vi "Test_PIL_Main.vi"() -> ()   [LabVIEW 2015]
uses:
  controls/EXPERIMENT_Inputs.ctl
  controls/LASER_Inputs.ctl
  controls/EXPERT_Inputs.ctl
  controls/SOFTWARE_Inputs.ctl
  controls/AO_6711_Inputs.ctl
  controls/AWG_5421_Inputs.ctl
  controls/DIGIT_5122_Inputs.ctl
  <instrlib>/niScope/Controls/niScope trigger source.ctl
  controls/HSDIO_6541_Inputs.ctl
  <instrlib>/niHSDIO/niHSDIO.llb/niHSDIO_ctl Trigger Source Values (Ring).ctl
  controls/VOLTAGES_Inputs.ctl
  controls/HEXA_Inputs.ctl
  controls/QUAD_Inputs.ctl
  controls/SEQUENCE_Inputs.ctl
  controls/TRAPPING_Inputs.ctl
  controls/EXCIT_Inputs.ctl
  controls/DATA_Inputs.ctl
  controls/TIMING_Inputs.ctl
  controls/SPECTRUM.ctl
  controls/QMH_UI_Cluster.ctl
  controls/QMH_UI_References.ctl
  controls/QMH_UI_Report.ctl
  controls/QMH_UI_Command.ctl
  controls/QMH_ICR_Command.ctl
  controls/QMH_Status.ctl
panel:
  out "données":dbl format="%.2f"
  in  "error in (no error)":errorcluster
  in  "Stop":bool
  in  "Start":bool
  in  "Save":bool
  in  "Load":bool
  in  "Exit":bool
  in  "Tabs":T1(tab)
  in  "SPECTRUM":T2={"Path of the Day"=path "D:/PIRENEA/DATA/2016/data_2016_01_01", "Spectrum Name"="2016_01_01_000.A00", "Accumulated"=FALSE, "Stored in Database"=FALSE, "Record Number"=0, "Quality Flag"="Optimal"}
  in  "Change Experiment":bool
  in  "EXPERIMENT Inputs":T3={"User Name"="", "Date"="", "Comment"="", "Experiment Steps"=[], "Sample Components"=[], "Molecules"=[], "Laser 1"={"Used"=TRUE, "Name"="Spectroscopy", "Reference"="Yag", "Wavelength"=1000.0, "Energy"=25.0}, "Laser 2"={"Used"=TRUE, "Name"="Spectroscopy", "Reference"="Yag", "Wavelength"=1000.0, "Energy"=25.0}, "Laser 3"={"Used"=TRUE, "Name"="Spectroscopy", "Reference"="Yag", "Wavelength"=1000.0, "Energy"=25.0}} caption="EXCIT Paths"
  in  "Change Voltages":bool
  in  "VOLTAGES Inputs":T5={"Hexa 1"={"Used"=FALSE, "Voltage"=0.0}, "Hexa 2"={"Used"=FALSE, "Voltage"=0.0}, "Hexa 3"={"Used"=FALSE, "Voltage"=0.0}, "Quad 1"={"Used"=TRUE, "Voltage"=25.0}, "Quad 2"={"Used"=TRUE, "Voltage"=25.0}, "Quad 3"={"Used"=TRUE, "Voltage"=25.0}}
  in  "SEQUENCE Inputs":T8={"TRAPPING Inputs"={"Init Values"=[], "Opening Values"=[0.0, 0.0, 0.0, 0.0], "Trapping Values"=[2.0, 5.0, 5.0, 2.0], "Emptying Values"=[-5.0, -5.0, -5.0, -5.0], "Adiabatic ON"=FALSE, "Adiabatic Duration"=1, "Adiabatic Waveforms"=["Adiabatic_None_2_2_2000.bin", "Adiabatic_Ramp_5_0_2000.bin", "Adiabatic_DoubleRamp_5_0_2000.bin", "Adiabatic_RC_2_0_2000.bin"]}, "EXCIT Inputs"={"Number of Excitations"=1, "Table of Waveforms"=[], "Script text"=""}, "DATA Inputs"={"Record Length"=0, "Sample Rate"=enum."20", "Number of Acquisitions"=1, "Type Of Data"=enum."I16", "Vertical Range"=enum."0.2"}, "TIMING Inputs"={"Number Of Acquisitions "=1, "Number Of Accumulations"=1, "Number Of Loops"=0, "Table of Waveforms"=[], "Script text"=""}} {"TIMING Inputs"."Number Of Loops" min=0 max=10; "TIMING Inputs"."Number Of Accumulations" min=0 max=50 step=1; "TIMING Inputs"."Number Of Acquisitions" min=1 max=10 step=1; "DATA Inputs"."Number of Acquisitions" min=1 max=10; "EXCIT Inputs"."Number of Excitations" min=1 max=10; "TRAPPING Inputs"."Trapping Values" min=-10.0 max=10.0; "TRAPPING Inputs"."Init Values" min=-10.0 max=10.0; "TRAPPING Inputs"."Emptying Values" min=-10.0 max=10.0; "TRAPPING Inputs"."Opening Values" min=-10.0 max=10.0}
  in  "Change Sequence":bool
  in  "Change Expert":bool
  in  "EXPERT Inputs":T13={"SOFTWARE Inputs"={"Application Directory"=path "D:/S.O.F.T.S/LABVIEW/PIL", "Resources Path"=path "D:/S.O.F.T.S/LABVIEW/PIL/resources", "Data Path"=path "D:/PIRENEA/DATA", "XML Path"=path "D:/PIRENEA/DATA", "XML File Filter"="*.xml", "Excit Scripts Path"=path "D:/PIRENEA/EXCIT_SCRIPTS", "Excit Scripts File Filter"="*.txt", "Excit Waveforms Path"=path "D:/PIRENEA/EXCIT_WFMS", "Excit Waveforms File Filter"="*.bin", "Timing Scripts Path"=path "D:/PIRENEA/SEQUENCE_SCRIPTS", "Timing Scripts File Filter"="*.txt", "Timing Waveforms Path"=path "D:/PIRENEA/SEQUENCE_WFMS", "Timing Waveforms File Filter"="*.bin", "Trapping Waveforms Path"=path "D:/PIRENEA/TRAPPING_WFMS", "Trapping Waveforms File Filter"="*.bin"}, "AO 6711 Inputs"={"Physical Channels"="AnalogOutput/ao0:3", "Min Voltage"=-10.0, "Max Voltage"=10.0, "Trigger Source"="/AnalogOutput/PFI0", "counter"="AnalogOutput/ctr0"}, "AWG 5421 Inputs"={"Resource Name"="WaveformGenerator", "Trigger Type"=2, "Trigger Source"="PFI0", "Sample Rate"=20000000.0}, "DIGIT 5122 Inputs"={"Sample Rate"=10000000.0, "Resource Name"="Digitizer", "Channel Name"="0", "Trigger Source"="VAL_EXTERNAL", "Vertical Range"=10.0, "Trigger Level"=3.0}, "HSDIO 6541 Inputs"={"Resource Name"="SequencerHSDIO", "Clock Rate"=1000000.0, "Trigger Source"="PFI0"}} {"HSDIO 6541 Inputs"."Clock Rate" format="%.2p"; "DIGIT 5122 Inputs"."Trigger Level" format="%.2f"; "DIGIT 5122 Inputs"."Vertical Range" format="%.2f"; "DIGIT 5122 Inputs"."Sample Rate" step=1000000.0 format="%.3p"; "AWG 5421 Inputs"."Sample Rate" format="%.2p"; "AWG 5421 Inputs"."Trigger Type" items=["None", "Software Edge", "Digital Edge", "Digital Level"]; "AO 6711 Inputs"."Max Voltage" min=-10.0 max=10.0; "AO 6711 Inputs"."Min Voltage" min=-10.0 max=10.0}
  out "QMH Status":string
  out "ICR Status":string
  out "QLA Status":string
  out "UI Status":string
  # "Name"
  # "Reference"
  # "(nm)"
  # "E (J)"
  # "Laser 1"
  # "Laser 2"
  # "Laser 3"
  # "HEXAPOLE"
  # "QUADRIPOLE"
  # "Gin"
  # "GI_in"
  # "GI_out"
  # "Gout"
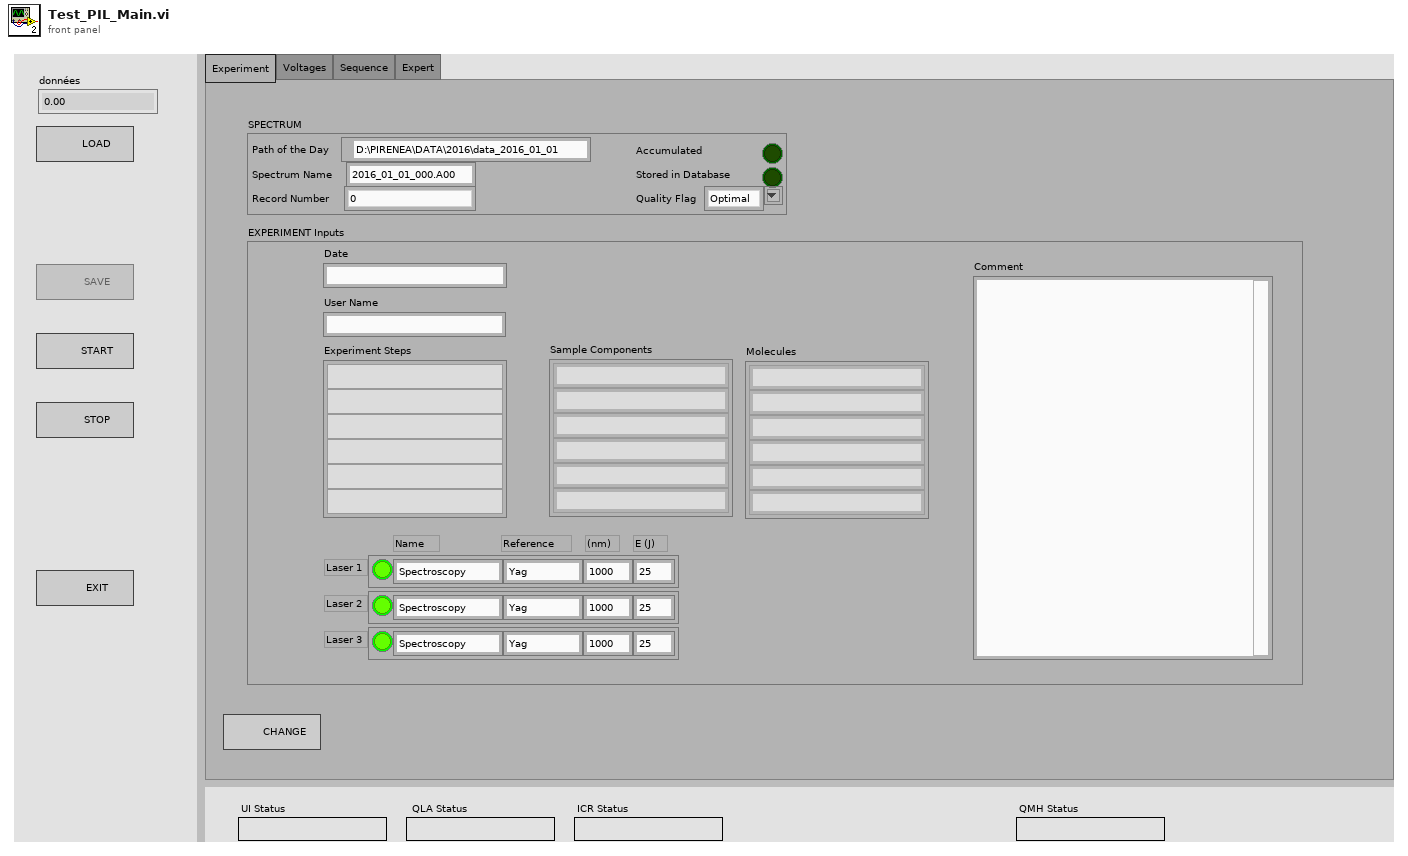
[diagram p1: front panel]
types:
  T1 = enum32{"Experiment", "Voltages", "Sequence", "Expert"}
  T2 = typedef "SPECTRUM.ctl" = cluster{"Path of the Day":path, "Spectrum Name":string, "Accumulated":bool, "Stored in Database":bool, "Record Number":i16, "Quality Flag":string}
  T3 = typedef "EXPERIMENT_Inputs.ctl" = cluster{"User Name":string, "Date":string, "Comment":string, "Experiment Steps":string[], "Sample Components":string[], "Molecules":string[], "Laser 1":T4, "Laser 2":T4, "Laser 3":T4}
  T4 = typedef "LASER_Inputs.ctl" = cluster{"Used":bool, "Name":string, "Reference":string, "Wavelength":dbl, "Energy":dbl}
  T5 = typedef "VOLTAGES_Inputs.ctl" = cluster{"Hexa 1":T6, "Hexa 2":T6, "Hexa 3":T6, "Quad 1":T7, "Quad 2":T7, "Quad 3":T7}
  T6 = typedef "HEXA_Inputs.ctl" = cluster{"Used":bool, "Voltage":dbl}
  T7 = typedef "QUAD_Inputs.ctl" = cluster{"Used":bool, "Voltage":dbl}
  T8 = typedef "SEQUENCE_Inputs.ctl" = cluster{"TRAPPING Inputs":T9, "EXCIT Inputs":T10, "DATA Inputs":T11, "TIMING Inputs":T12}
  T9 = typedef "TRAPPING_Inputs.ctl" = cluster{"Init Values":dbl[], "Opening Values":dbl[], "Trapping Values":dbl[], "Emptying Values":dbl[], "Adiabatic ON":bool, "Adiabatic Duration":i32, "Adiabatic Waveforms":string[]}
  T10 = typedef "EXCIT_Inputs.ctl" = cluster{"Number of Excitations":i32, "Table of Waveforms":string[], "Script text":string}
  T11 = typedef "DATA_Inputs.ctl" = cluster{"Record Length":i32, "Sample Rate":enum16{"1", "2", "5", "10", "20", "25", "50", "100"}, "Number of Acquisitions":i32, "Type Of Data":enum16{"I16", "DBL"}, "Vertical Range":enum16{"0.2", "0.4", "1", "2", "4", "10"}}
  T12 = typedef "TIMING_Inputs.ctl" = cluster{"Number Of Acquisitions ":i16, "Number Of Accumulations":i16, "Number Of Loops":i16, "Table of Waveforms":string[], "Script text":string}
  T13 = typedef "EXPERT_Inputs.ctl" = cluster{"SOFTWARE Inputs":T14, "AO 6711 Inputs":T15, "AWG 5421 Inputs":T16, "DIGIT 5122 Inputs":T17, "HSDIO 6541 Inputs":T19}
  T14 = typedef "SOFTWARE_Inputs.ctl" = cluster{"Application Directory":path, "Resources Path":path, "Data Path":path, "XML Path":path, "XML File Filter":string, "Excit Scripts Path":path, "Excit Scripts File Filter":string, "Excit Waveforms Path":path, "Excit Waveforms File Filter":string, "Timing Scripts Path":path, "Timing Scripts File Filter":string, "Timing Waveforms Path":path, "Timing Waveforms File Filter":string, "Trapping Waveforms Path":path, "Trapping Waveforms File Filter":string}
  T15 = typedef "AO_6711_Inputs.ctl" = cluster{"Physical Channels":tag, "Min Voltage":dbl, "Max Voltage":dbl, "Trigger Source":tag, "counter":tag}
  T16 = typedef "AWG_5421_Inputs.ctl" = cluster{"Resource Name":refnum<k15>, "Trigger Type":u16, "Trigger Source":string, "Sample Rate":dbl}
  T17 = typedef "DIGIT_5122_Inputs.ctl" = cluster{"Sample Rate":dbl, "Resource Name":refnum<k15>, "Channel Name":string, "Trigger Source":T18, "Vertical Range":dbl, "Trigger Level":dbl}
  T18 = typedef "niScope trigger source.ctl" = string
  T19 = typedef "HSDIO_6541_Inputs.ctl" = cluster{"Resource Name":refnum<k15>, "Clock Rate":dbl, "Trigger Source":T20}
  T20 = typedef "niHSDIO_ctl Trigger Source Values (Ring).ctl" = string
  T21 = typedef "QMH_UI_Cluster.ctl" = cluster{"QMH UI References":T22, "QMH UI Report":T23}
  T22 = typedef "QMH_UI_References.ctl" = cluster{"Refnum Load":refnum<vi>, "Refnum Save":refnum<vi>, "Refnum Start":refnum<vi>, "Refnum Stop":refnum<vi>, "Refnum Exit":refnum<vi>, "Refnum Tabs":refnum<vi>, "Refnum SPECTRUM":refnum<vi>, "Refnum EXPERIMENT":refnum<vi>, "Refnum VOLTAGES":refnum<vi>, "Refnum SEQUENCE":refnum<vi>, "Refnum EXPERT":refnum<vi>, "Refnum CHANGE Experiment":refnum<vi>, "Refnum CHANGE Voltages":refnum<vi>, "Refnum CHANGE Sequence":refnum<vi>, "Refnum CHANGE Expert":refnum<vi>}
  T23 = typedef "QMH_UI_Report.ctl" = cluster{"UI Status":T24, "QLA Status":string, "ICR Status":T25, "QMH Status":T26}
  T24 = typedef "QMH_UI_Command.ctl" = enum16{"Initialize", "UI Load", "UI Save", "UI Change Experiment", "UI Change Voltages", "UI Change Sequence", "UI Change Expert", "Ready to Start", "UI Start", "UI Stop", "UI Exit", "Update Report", "Update ICR Report"}
  T25 = typedef "QMH_ICR_Command.ctl" = enum16{"Initialize", "Hardware Setup", "Waiting for Trigger", "Sequence Started", "Sequence Finished", "Writing Data", "Hardware Reset", "Exit"}
  T26 = typedef "QMH_Status.ctl" = enum16{"Init", "Loading", "Setup", "Ready to Start", "Started", "Idle"}
  T27 = typedef "QMH_UI_Message.ctl" = cluster{"Command":T24, "Data":variant}
  T28 = enum32{"invalid app kind", "Development System", "Run Time System", "Student Edition", "Embedded LabVIEW", "Evaluation", "Custom"}
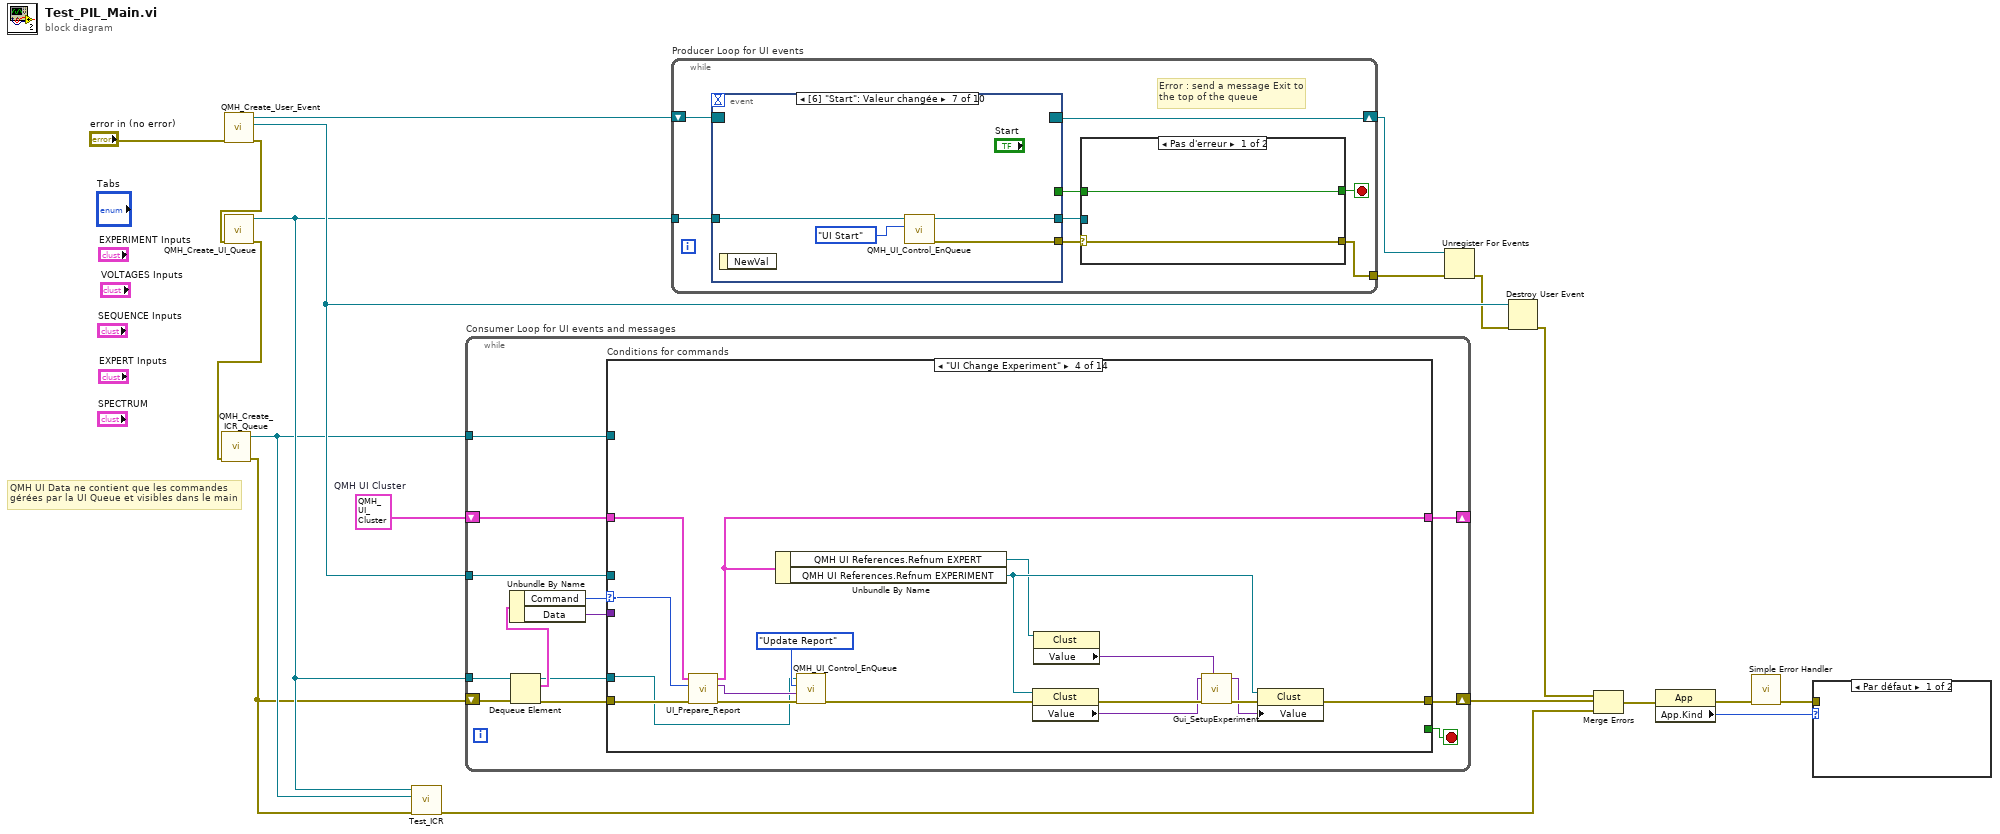
[diagram p0: block diagram]
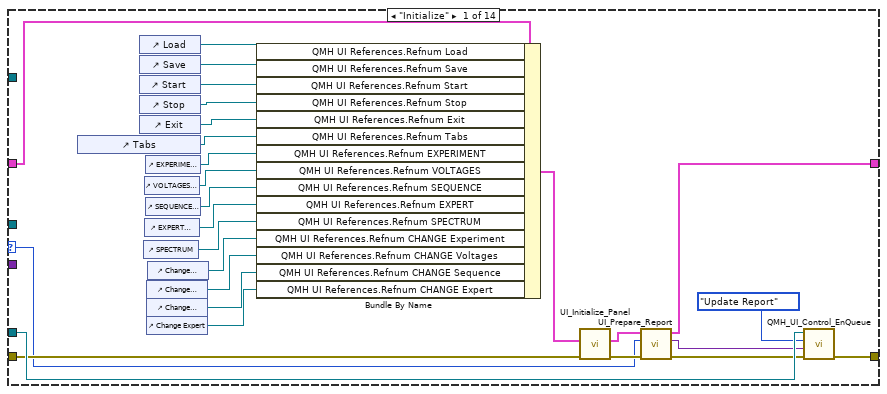
[diagram p2: hidden frame]
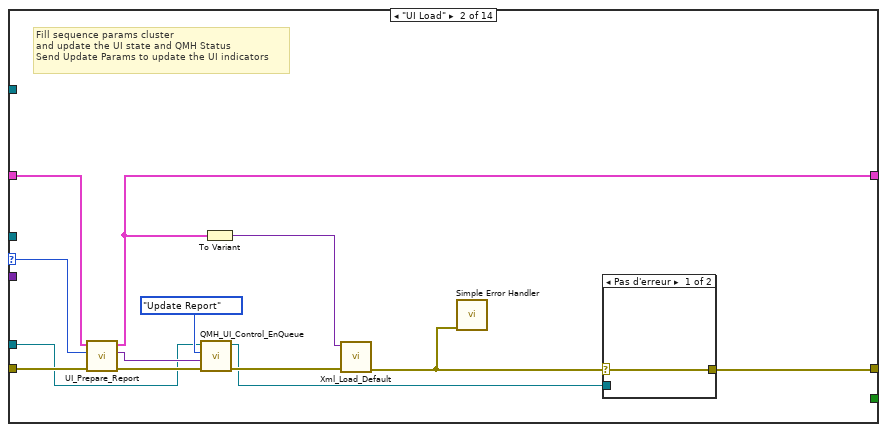
[diagram p3: hidden frame]
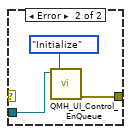
[diagram p4: hidden frame]
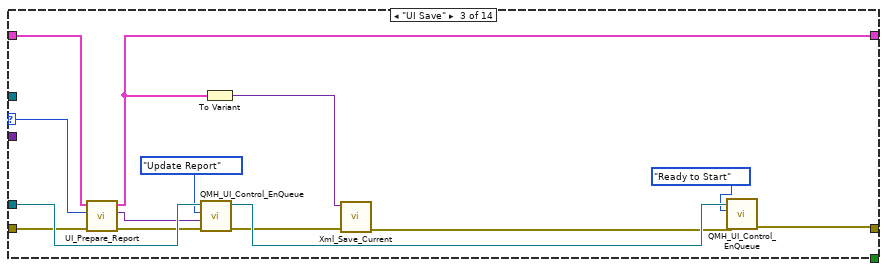
[diagram p5: hidden frame]
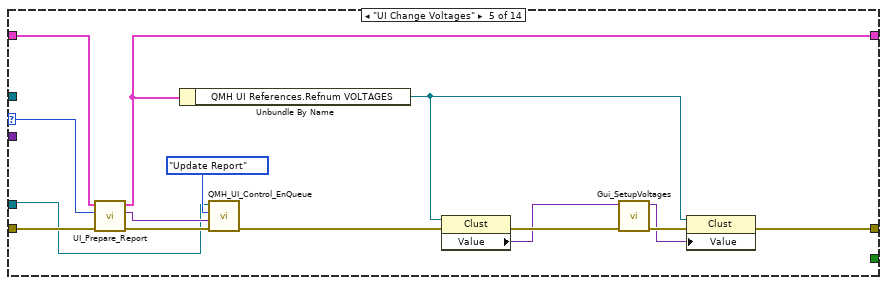
[diagram p6: hidden frame]
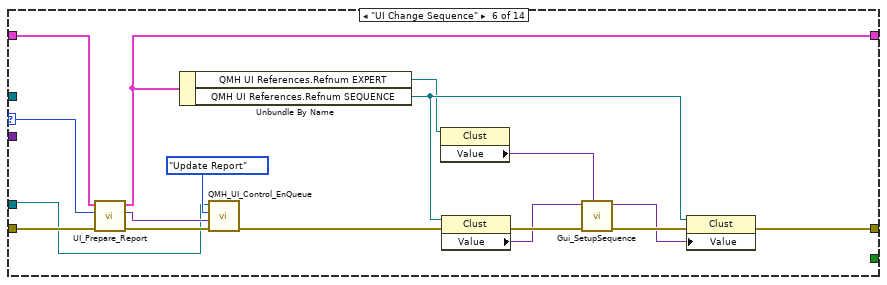
[diagram p7: hidden frame]
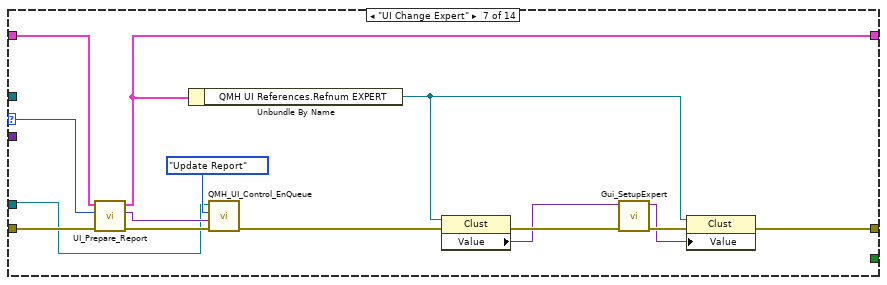
[diagram p8: hidden frame]
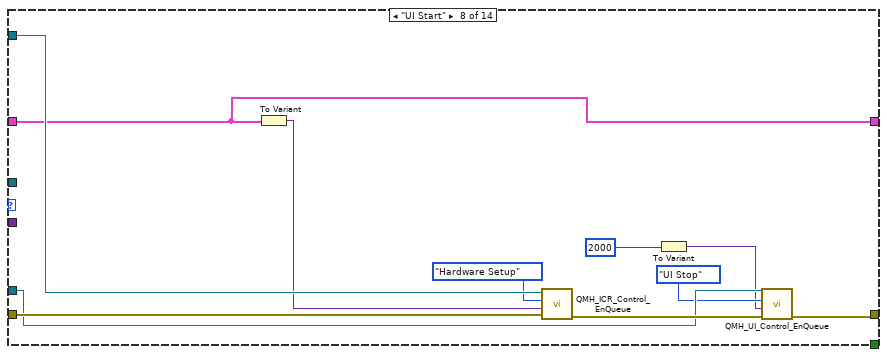
[diagram p9: hidden frame]
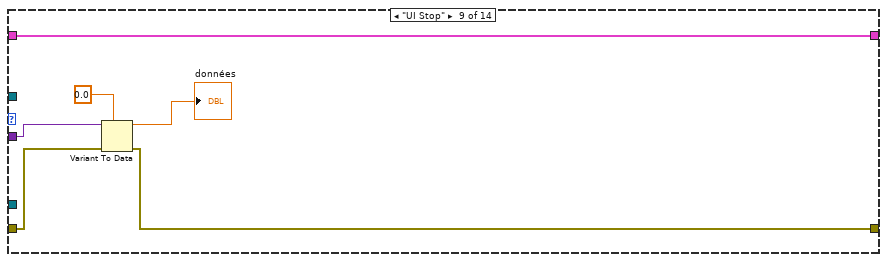
[diagram p10: hidden frame]
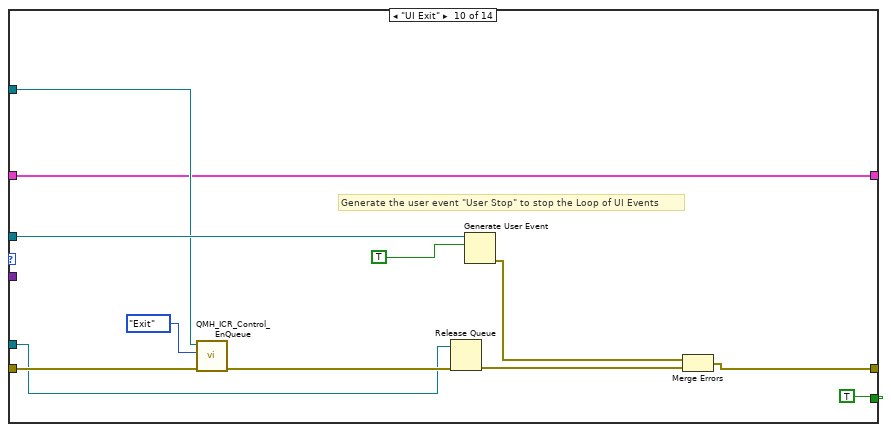
[diagram p11: hidden frame]
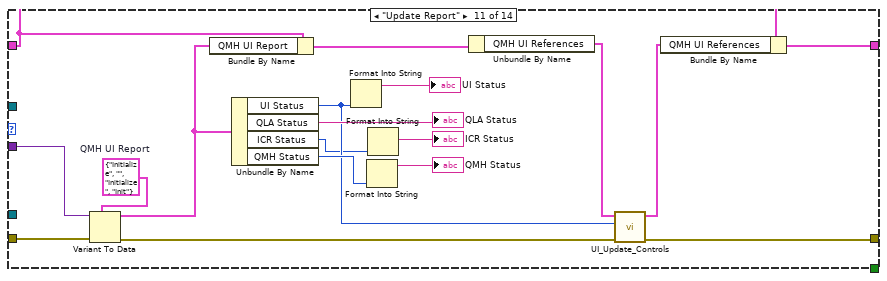
[diagram p12: hidden frame]
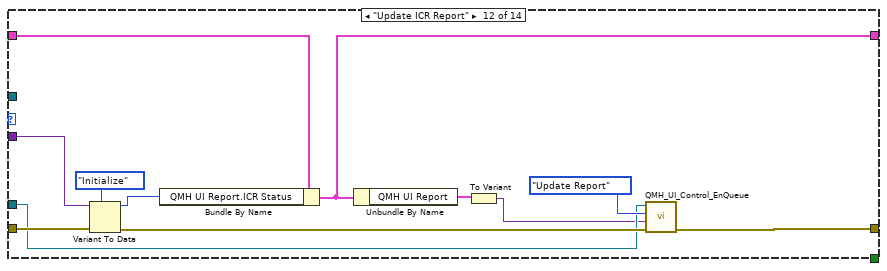
[diagram p13: hidden frame]
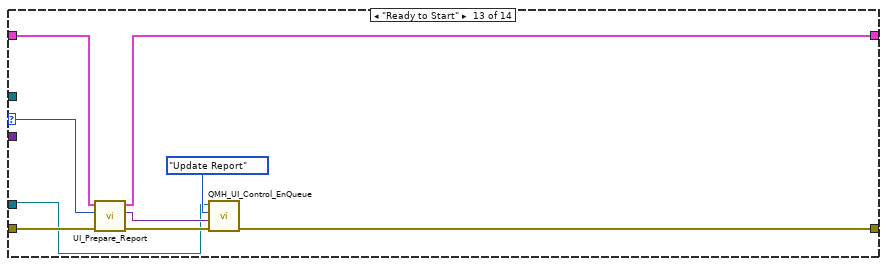
[diagram p14: hidden frame]
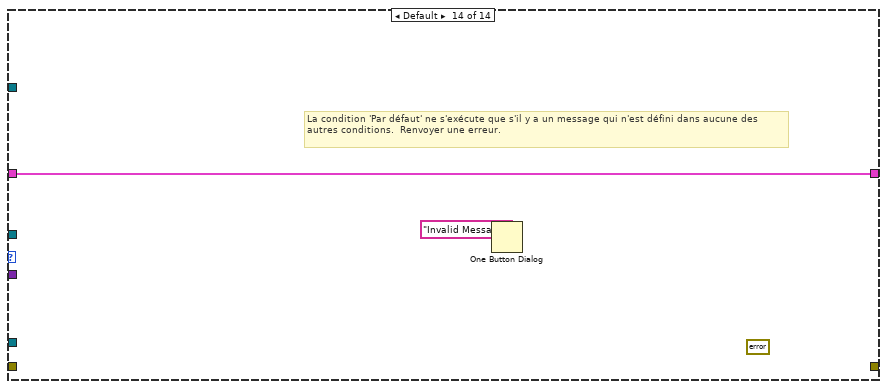
[diagram p15: hidden frame]
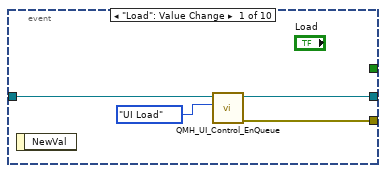
[diagram p16: hidden frame]
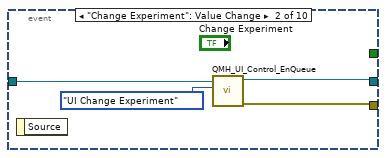
[diagram p17: hidden frame]
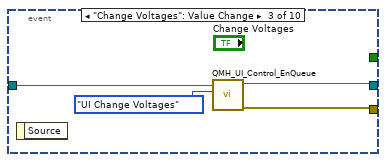
[diagram p18: hidden frame]
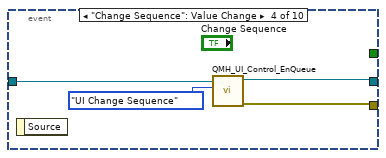
[diagram p19: hidden frame]
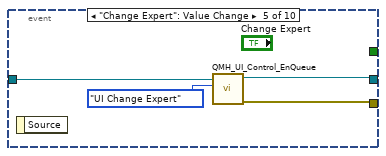
[diagram p20: hidden frame]
diagram:
  w18 = T21 {"QMH UI References"={"Refnum Load"=refnum, "Refnum Save"=refnum, "Refnum Start"=refnum, "Refnum Stop"=refnum, "Refnum Exit"=refnum, "Refnum Tabs"=refnum, "Refnum SPECTRUM"=refnum, "Refnum EXPERIMENT"=refnum, "Refnum VOLTAGES"=refnum, "Refnum SEQUENCE"=refnum, "Refnum EXPERT"=refnum, "Refnum CHANGE Experiment"=refnum, "Refnum CHANGE Voltages"=refnum, "Refnum CHANGE Sequence"=refnum, "Refnum CHANGE Expert"=refnum}, "QMH UI Report"={"UI Status"=enum."Initialize", "QLA Status"="", "ICR Status"=enum."Initialize", "QMH Status"=enum."Init"}}  # QMH UI Cluster
  # "QMH UI Data ne contient que les commandes\ngérées par la UI Queue et visibles dans le main"
  n1 = call "QMH_Create_User_Event.vi"("error in (no error)"="error in (no error)") -> ("error out"=w16:errorcluster, "User Stop Event"=w12:refnum<user-event>, "Refnum register for events"=w19:refnum<event-registration>)  [unwired: 8 in]
  n2 = call "QMH_Create_UI_Queue.vi"("error in (no error)"=w16) -> ("error out"=w2:errorcluster, "UI Queue"=w5:refnum<queue>)  [unwired: 9 in]
  n3 = call "QMH_Create_ICR_Queue.vi"("error in (no error)"=w2) -> ("error out"=w1:errorcluster, "ICR Queue"=w4:refnum<queue>)  [unwired: 9 in]
  n4 = call "Test_ICR.vi"("error in (no error)"=w1, "ICR Queue"=w4, "UI Queue"=w5) -> ("error out"=w3:errorcluster)  [unwired: 8 in]
  n5 = while "Consumer Loop for UI events and messages" {
    shift-right: [w23] -> _
    shift-left: w18 -> [w32]
    shift-right: [w21] -> w13
    shift-left: w1 -> [w28]
    tunnel: w5 -> [w29]
    tunnel: w12 -> [w24]
    tunnel: w4 -> [w20]
    stop <- w31 stop-if-true
    n6 = Dequeue Element(queue=w29, error in (no error)=w28) -> (queue out=w27:refnum<queue>, element=w30:T27, error out=w22:errorcluster)  [unwired: 2 out]
    n7 = Unbundle By Name(w30) -> ("Command"=w26:T24, "Data"=w25:variant)
    n8 = case "Conditions for commands" shown="\"UI Change Experiment\"" w26 {
      selector: w26 -> [w39 w69 w86 w102 w117 w134 w149 _ _ _ _ _ w218 _]
      tunnel: w27 -> [w53 w62 w90 w100 w115 w132 w147 w161 _ w174 _ w205 w216 _]
      tunnel: w32 -> [w54 w68 w85 w103 w118 w135 w150 w157 w166 w172 w186 w211 w219 w223]
      tunnel: [_ _ _ _ _ _ _ _ _ TRUE _ _ _ _] -> w31
      tunnel: w25 -> [_ _ _ _ _ _ _ _ w171 _ w201 w213 _ _]
      tunnel: w24 -> [_ _ _ _ _ _ _ _ _ w180 _ _ _ _]
      tunnel: [w40 w65 w79 w99 w114 w131 w146 w157 w166 w172 w196 w202 w215 w223] -> w23
      tunnel: w22 -> [w45 w70 w87 w101 w116 w133 w148 w165 w168 w176 w193 w212 w217 _]
      tunnel: [w38 w63 w82 w91 w108 w125 w140 w162 w167 w178 w192 w206 w214 _] -> w21
      tunnel: w20 -> [_ _ _ _ _ _ _ w164 _ w173 _ _ _ _]
      frame "Initialize" {
        n9 = control-ref of="Tabs"() -> (w50:refnum<vi>)
        n10 = control-ref of="Load"() -> (w59:refnum<vi>)
        n11 = control-ref of="Save"() -> (w58:refnum<vi>)
        n12 = control-ref of="Start"() -> (w57:refnum<vi>)
        n13 = control-ref of="Stop"() -> (w56:refnum<vi>)
        n14 = control-ref of="Exit"() -> (w55:refnum<vi>)
        n15 = control-ref of="SPECTRUM"() -> (w37:refnum<vi>)
        n16 = control-ref of="VOLTAGES Inputs"() -> (w48:refnum<vi>)
        n17 = control-ref of="EXPERT Inputs"() -> (w46:refnum<vi>)
        n18 = control-ref of="EXPERIMENT Inputs"() -> (w49:refnum<vi>)
        n19 = control-ref of="SEQUENCE Inputs"() -> (w47:refnum<vi>)
        n20 = control-ref of="Change Voltages"() -> (w33:refnum<vi>)
        n21 = control-ref of="Change Sequence"() -> (w34:refnum<vi>)
        n22 = control-ref of="Change Expert"() -> (w35:refnum<vi>)
        n23 = control-ref of="Change Experiment"() -> (w36:refnum<vi>)
        n24 = Bundle By Name(cluster=w54, "QMH UI References.Refnum Load"=w59, "QMH UI References.Refnum Save"=w58, "QMH UI References.Refnum Start"=w57, "QMH UI References.Refnum Stop"=w56, "QMH UI References.Refnum Exit"=w55, "QMH UI References.Refnum Tabs"=w50, "QMH UI References.Refnum EXPERIMENT"=w49, "QMH UI References.Refnum VOLTAGES"=w48, "QMH UI References.Refnum SEQUENCE"=w47, "QMH UI References.Refnum EXPERT"=w46, "QMH UI References.Refnum SPECTRUM"=w37, "QMH UI References.Refnum CHANGE Experiment"=w36, "QMH UI References.Refnum CHANGE Voltages"=w33, "QMH UI References.Refnum CHANGE Sequence"=w34, "QMH UI References.Refnum CHANGE Expert"=w35) -> (w51:T21)
        n25 = call "UI_Initialize_Panel.vi"("error in (no error)"=w45, "QMH UI Cluster"=w51) -> ("error out"=w44:errorcluster, "QMH UI Cluster"=w41:T21)  [unwired: 8 in]
        n26 = call "UI_Prepare_Report.vi"("error in (no error)"=w44, "UI Status"=w39, "QMH UI Cluster"=w41) -> ("error out"=w43:errorcluster, "Variant"=w42:variant, "QMH UI Cluster"=w40:T21)  [unwired: 6 in]
        n27 = call "QMH_UI_Control_EnQueue.vi"("error in (no error)"=w43, "Variant"=w42, "Command"=QMH_UI_Command."Update Report", "UI Queue"=w53) -> ("error out"=w38:errorcluster)  [unwired: 6 in, 1 out]
      }
      frame "UI Load" {
        # "Fill sequence params cluster\nand update the UI state and QMH Status\nSend Update Params to update the UI indicators"
        n28 = call "UI_Prepare_Report.vi"("error in (no error)"=w70, "UI Status"=w69, "QMH UI Cluster"=w68) -> ("error out"=w71:errorcluster, "Variant"=w67:variant, "QMH UI Cluster"=w65:T21)  [unwired: 6 in]
        n29 = call "QMH_UI_Control_EnQueue.vi"("error in (no error)"=w71, "Variant"=w67, "Command"=QMH_UI_Command."Update Report", "UI Queue"=w62) -> ("error out"=w66:errorcluster, "UI Queue"=w61:refnum<queue>)  [unwired: 6 in]
        n30 = To Variant(anything=w65) -> (Variant=w64:variant)
        n31 = call "Xml_Load_Default.vi"("error in (no error)"=w66, "Variant"=w64) -> ("error out"=w60:errorcluster)  [unwired: 9 in]
        n32 = call <vilib>:"Simple Error Handler.vi"("error in (no error)"=w60) -> ()  [unwired: 4 in, 5 out]
        n33 = case shown="Pas d'erreur" w60 {
          selector: w60 -> [w73 _]
          tunnel: [w73 w76] -> w63
          tunnel: w61 -> [_ w74]
          frame No Error {
          }
          frame Error {
            n34 = call "QMH_UI_Control_EnQueue.vi"("Command"=QMH_UI_Command."Initialize", "UI Queue"=w74) -> ("error out"=w76:errorcluster)  [unwired: 8 in, 1 out]
          }
        }
      }
      frame "UI Save" {
        n35 = call "UI_Prepare_Report.vi"("error in (no error)"=w87, "UI Status"=w86, "QMH UI Cluster"=w85) -> ("error out"=w88:errorcluster, "Variant"=w84:variant, "QMH UI Cluster"=w79:T21)  [unwired: 6 in]
        n36 = call "QMH_UI_Control_EnQueue.vi"("error in (no error)"=w88, "Variant"=w84, "Command"=QMH_UI_Command."Update Report", "UI Queue"=w90) -> ("error out"=w80:errorcluster, "UI Queue"=w83:refnum<queue>)  [unwired: 6 in]
        n37 = To Variant(anything=w79) -> (Variant=w78:variant)
        n38 = call "Xml_Save_Current.vi"("error in (no error)"=w80, "Variant"=w78) -> ("error out"=w77:errorcluster)  [unwired: 9 in]
        n39 = call "QMH_UI_Control_EnQueue.vi"("error in (no error)"=w77, "Command"=QMH_UI_Command."Ready to Start", "UI Queue"=w83) -> ("error out"=w82:errorcluster)  [unwired: 7 in, 1 out]
      }
      frame "UI Change Experiment" {
        n40 = call "UI_Prepare_Report.vi"("error in (no error)"=w101, "UI Status"=w102, "QMH UI Cluster"=w103) -> ("error out"=w105:errorcluster, "Variant"=w104:variant, "QMH UI Cluster"=w99:T21)  [unwired: 6 in]
        n41 = Unbundle By Name(w99) -> ("QMH UI References.Refnum EXPERT"=w93:refnum<vi>, "QMH UI References.Refnum EXPERIMENT"=w98:refnum<vi>)
        n42 = call "QMH_UI_Control_EnQueue.vi"("error in (no error)"=w105, "Variant"=w104, "Command"=QMH_UI_Command."Update Report", "UI Queue"=w100) -> ("error out"=w97:errorcluster)  [unwired: 6 in, 1 out]
        n43 = property class="Clust"(reference=w98, error in=w97) -> (error out=w96:errorcluster, "Value"=w95:variant)  [unwired: 1 out]
        n44 = property class="Clust"(reference=w93) -> ("Value"=w92:variant)  [unwired: 1 in, 2 out]
        n45 = call "Gui_SetupExperiment.vi"("Variant for Path"=w92, "error in (no error)"=w96, "Variant"=w95) -> ("error out"=w107:errorcluster, "Variant Output"=w94:variant)  [unwired: 7 in]
        n46 = property class="Clust"(reference=w98, error in=w107, "Value"=w94) -> (error out=w91:errorcluster)  [unwired: 1 out]
      }
      frame "UI Change Voltages" {
        n47 = call "UI_Prepare_Report.vi"("error in (no error)"=w116, "UI Status"=w117, "QMH UI Cluster"=w118) -> ("error out"=w120:errorcluster, "Variant"=w119:variant, "QMH UI Cluster"=w114:T21)  [unwired: 6 in]
        n48 = Unbundle By Name(w114) -> ("QMH UI References.Refnum VOLTAGES"=w113:refnum<vi>)
        n49 = call "QMH_UI_Control_EnQueue.vi"("error in (no error)"=w120, "Variant"=w119, "Command"=QMH_UI_Command."Update Report", "UI Queue"=w115) -> ("error out"=w112:errorcluster)  [unwired: 6 in, 1 out]
        n50 = property class="Clust"(reference=w113, error in=w112) -> (error out=w111:errorcluster, "Value"=w110:variant)  [unwired: 1 out]
        n51 = call "Gui_SetupVoltages.vi"("error in (no error)"=w111, "Variant"=w110) -> ("error out"=w122:errorcluster, "Variant Output"=w109:variant)  [unwired: 8 in]
        n52 = property class="Clust"(reference=w113, error in=w122, "Value"=w109) -> (error out=w108:errorcluster)  [unwired: 1 out]
      }
      frame "UI Change Sequence" {
        n53 = call "UI_Prepare_Report.vi"("error in (no error)"=w133, "UI Status"=w134, "QMH UI Cluster"=w135) -> ("error out"=w137:errorcluster, "Variant"=w136:variant, "QMH UI Cluster"=w131:T21)  [unwired: 6 in]
        n54 = Unbundle By Name(w131) -> ("QMH UI References.Refnum EXPERT"=w124:refnum<vi>, "QMH UI References.Refnum SEQUENCE"=w130:refnum<vi>)
        n55 = call "QMH_UI_Control_EnQueue.vi"("error in (no error)"=w137, "Variant"=w136, "Command"=QMH_UI_Command."Update Report", "UI Queue"=w132) -> ("error out"=w129:errorcluster)  [unwired: 6 in, 1 out]
        n56 = property class="Clust"(reference=w124) -> ("Value"=w123:variant)  [unwired: 1 in, 2 out]
        n57 = property class="Clust"(reference=w130, error in=w129) -> (error out=w128:errorcluster, "Value"=w127:variant)  [unwired: 1 out]
        n58 = call "Gui_SetupSequence.vi"("Variant For Path"=w123, "error in (no error)"=w128, "Variant"=w127) -> ("error out"=w139:errorcluster, "Variant Output"=w126:variant)  [unwired: 7 in]
        n59 = property class="Clust"(reference=w130, error in=w139, "Value"=w126) -> (error out=w125:errorcluster)  [unwired: 1 out]
      }
      frame "UI Change Expert" {
        n60 = call "UI_Prepare_Report.vi"("error in (no error)"=w148, "UI Status"=w149, "QMH UI Cluster"=w150) -> ("error out"=w152:errorcluster, "Variant"=w151:variant, "QMH UI Cluster"=w146:T21)  [unwired: 6 in]
        n61 = Unbundle By Name(w146) -> ("QMH UI References.Refnum EXPERT"=w145:refnum<vi>)
        n62 = call "QMH_UI_Control_EnQueue.vi"("error in (no error)"=w152, "Variant"=w151, "Command"=QMH_UI_Command."Update Report", "UI Queue"=w147) -> ("error out"=w144:errorcluster)  [unwired: 6 in, 1 out]
        n63 = property class="Clust"(reference=w145, error in=w144) -> (error out=w143:errorcluster, "Value"=w142:variant)  [unwired: 1 out]
        n64 = call "Gui_SetupExpert.vi"("error in (no error)"=w143, "Variant"=w142) -> ("error out"=w154:errorcluster, "Variant Output"=w141:variant)  [unwired: 8 in]
        n65 = property class="Clust"(reference=w145, error in=w154, "Value"=w141) -> (error out=w140:errorcluster)  [unwired: 1 out]
      }
      frame "UI Start" {
        n66 = To Variant(anything=w157) -> (Variant=w155:variant)
        n67 = call "QMH_ICR_Control_EnQueue.vi"("error in (no error)"=w165, "Variant"=w155, "Command"=QMH_ICR_Command."Hardware Setup", "ICR Queue"=w164) -> ("error out"=w163:errorcluster)  [unwired: 6 in, 1 out]
        n68 = To Variant(anything=2000) -> (Variant=w159:variant)
        n69 = call "QMH_UI_Control_EnQueue.vi"("error in (no error)"=w163, "Variant"=w159, "Command"=QMH_UI_Command."UI Stop", "UI Queue"=w161) -> ("error out"=w162:errorcluster)  [unwired: 6 in, 1 out]
      }
      frame "UI Stop" {
        n70 = Variant To Data(error in=w168, type=0.0, Variant=w171) -> (data=→"données":dbl, error out=w167:errorcluster)
      }
      frame "UI Exit" {
        # "Generate the user event \"User Stop\" to stop the Loop of UI Events"
        n71 = call "QMH_ICR_Control_EnQueue.vi"("error in (no error)"=w176, "Command"=QMH_ICR_Command."Exit", "ICR Queue"=w173) -> ("error out"=w175:errorcluster)  [unwired: 7 in, 1 out]
        n72 = Release Queue(queue=w174, error in (no error)=w175) -> (error out=w182:errorcluster)  [unwired: 1 in, 2 out]
        n73 = Generate User Event(user event=w180, event data cluster=TRUE ("données d'événement")) -> (error out=w179:errorcluster)  [unwired: 2 in, 1 out]
        n74 = Merge Errors(w179, w182) -> (w178:errorcluster)
      }
      frame "Update Report" {
        w200 = T23 {"UI Status"=enum."Initialize", "QLA Status"="", "ICR Status"=enum."Initialize", "QMH Status"=enum."Init"}  # QMH UI Report
        n75 = Variant To Data(error in=w193, type=w200, Variant=w201) -> (data=w188:T23, error out=w198:errorcluster)
        n76 = Bundle By Name(cluster=w186, "QMH UI Report"=w188) -> (w187:T21)
        n77 = Unbundle By Name(w188) -> ("UI Status"=w190:T24, "QLA Status"=→"QLA Status":string, "ICR Status"=w185:T25, "QMH Status"=w194:T26)
        n78 = Format Into String ("Format to String")(w190) -> (resulting string=→"UI Status":string)  [unwired: 3 in, 1 out]
        n79 = Format Into String ("Format to String")(w194) -> (resulting string=→"QMH Status":string)  [unwired: 3 in, 1 out]
        n80 = Format Into String ("Format to String")(w185) -> (resulting string=→"ICR Status":string)  [unwired: 3 in, 1 out]
        n81 = Unbundle By Name(w187) -> ("QMH UI References"=w189:T22)
        n82 = call "UI_Update_Controls.vi"("error in (no error)"=w198, "UI Status"=w190, "QMH UI References"=w189) -> ("error out"=w192:errorcluster, "QMH UI References"=w197:T22)  [unwired: 7 in]
        n83 = Bundle By Name(cluster=w186, "QMH UI References"=w197) -> (w196:T21)
      }
      frame "Update ICR Report" {
        n84 = Variant To Data(error in=w212, type=QMH_ICR_Command."Initialize" ("Command"), Variant=w213) -> (data=w209:T25, error out=w207:errorcluster)
        n85 = Bundle By Name(cluster=w211, "QMH UI Report.ICR Status"=w209) -> (w202:T21)
        n86 = Unbundle By Name(w202) -> ("QMH UI Report"=w203:T23)
        n87 = To Variant(anything=w203) -> (Variant=w204:variant)
        n88 = call "QMH_UI_Control_EnQueue.vi"("error in (no error)"=w207, "Variant"=w204, "Command"=QMH_UI_Command."Update Report", "UI Queue"=w205) -> ("error out"=w206:errorcluster)  [unwired: 6 in, 1 out]
      }
      frame "Ready to Start" {
        n89 = call "UI_Prepare_Report.vi"("error in (no error)"=w217, "UI Status"=w218, "QMH UI Cluster"=w219) -> ("error out"=w221:errorcluster, "Variant"=w220:variant, "QMH UI Cluster"=w215:T21)  [unwired: 6 in]
        n90 = call "QMH_UI_Control_EnQueue.vi"("error in (no error)"=w221, "Variant"=w220, "Command"=QMH_UI_Command."Update Report", "UI Queue"=w216) -> ("error out"=w214:errorcluster)  [unwired: 6 in, 1 out]
      }
      frame Default {
        (unwired) errorcluster {"status"=FALSE, "code"=0, "source"=""} ("sortie d'erreur")
        # "La condition 'Par défaut' ne s'exécute que s'il y a un message qui n'est défini dans aucune des autres conditions.  Renvoyer une erreur."
        n91 = One Button Dialog(message="Invalid Message") -> ()  [unwired: 1 in, 1 out]
      }
    }
  }
  n92 = while "Producer Loop for UI events" {
    tunnel: w5 -> [w231]
    tunnel: [w225] -> w15
    shift-right: [w227] -> w14
    shift-left: w19 -> [w228]
    stop <- w232 stop-if-true
    # "Error : send a message Exit to\nthe top of the queue"
    n93 = event shown="[6] \"Start\": Valeur changée" {
      selector: w228 -> [_ _ _ _ _ _ _ _ _ _]
      dyn-events: [_ _ _ _ _ _ _ _ _ _] -> w227
      timeout: _ -> [_ _ _ _ _ _ _ _ _ _]
      tunnel: w231 -> [w235 w237 w241 w245 w249 w255 w259 w263 w268 w270]
      tunnel: [w233 w238 w242 w246 w250 w253 w257 w261 w267 _] -> w230
      tunnel: [w234 w239 w243 w247 w251 w254 w258 w262 w266 w270] -> w229
      tunnel: [_ _ _ _ _ _ _ _ _ TRUE ("User Stop")] -> w226
      event "Load": Value Change {
        n94 = event-data() -> ()  [unwired: 2 out]
        n95 = call "QMH_UI_Control_EnQueue.vi"("Command"=QMH_UI_Command."UI Load", "UI Queue"=w235) -> ("error out"=w233:errorcluster, "UI Queue"=w234:refnum<queue>)  [unwired: 8 in]
      }
      event "Change Experiment": Value Change {
        n96 = event-data() -> ()  [unwired: 2 out]
        n97 = call "QMH_UI_Control_EnQueue.vi"("Command"=QMH_UI_Command."UI Change Experiment", "UI Queue"=w237) -> ("error out"=w238:errorcluster, "UI Queue"=w239:refnum<queue>)  [unwired: 8 in]
      }
      event "Change Voltages": Value Change {
        n98 = event-data() -> ()  [unwired: 2 out]
        n99 = call "QMH_UI_Control_EnQueue.vi"("Command"=QMH_UI_Command."UI Change Voltages", "UI Queue"=w241) -> ("error out"=w242:errorcluster, "UI Queue"=w243:refnum<queue>)  [unwired: 8 in]
      }
      event "Change Sequence": Value Change {
        n100 = event-data() -> ()  [unwired: 2 out]
        n101 = call "QMH_UI_Control_EnQueue.vi"("Command"=QMH_UI_Command."UI Change Sequence", "UI Queue"=w245) -> ("error out"=w246:errorcluster, "UI Queue"=w247:refnum<queue>)  [unwired: 8 in]
      }
      event "Change Expert": Value Change {
        n102 = event-data() -> ()  [unwired: 2 out]
        n103 = call "QMH_UI_Control_EnQueue.vi"("Command"=QMH_UI_Command."UI Change Expert", "UI Queue"=w249) -> ("error out"=w250:errorcluster, "UI Queue"=w251:refnum<queue>)  [unwired: 8 in]
      }
      event "Save": Value Change {
        n104 = event-data() -> ()  [unwired: 2 out]
        n105 = call "QMH_UI_Control_EnQueue.vi"("Command"=QMH_UI_Command."UI Save", "UI Queue"=w255) -> ("error out"=w253:errorcluster, "UI Queue"=w254:refnum<queue>)  [unwired: 8 in]
      }
      event "Start": Value Change {
        n106 = event-data() -> ()  [unwired: 2 out]
        n107 = call "QMH_UI_Control_EnQueue.vi"("Command"=QMH_UI_Command."UI Start", "UI Queue"=w259) -> ("error out"=w257:errorcluster, "UI Queue"=w258:refnum<queue>)  [unwired: 8 in]
      }
      event "Stop": Value Change {
        n108 = event-data() -> ()  [unwired: 2 out]
        n109 = call "QMH_UI_Control_EnQueue.vi"("Command"=QMH_UI_Command."UI Stop", "UI Queue"=w263) -> ("error out"=w261:errorcluster, "UI Queue"=w262:refnum<queue>)  [unwired: 8 in]
      }
      event "Exit": Value Change {
        n110 = event-data() -> ()  [unwired: 2 out]
        n111 = call "QMH_UI_Control_EnQueue.vi"("Command"=QMH_UI_Command."UI Exit", "UI Queue"=w268) -> ("error out"=w267:errorcluster, "UI Queue"=w266:refnum<queue>)  [unwired: 8 in]
      }
      event User Event {
        n112 = event-data() -> ()  [unwired: 3 out]
      }
    }
    n113 = case shown="Pas d'erreur" w230 {
      selector: w230 -> [w271 _]
      tunnel: [w272 TRUE] -> w232
      tunnel: w229 -> [_ w276]
      tunnel: w226 -> [w272 _]
      tunnel: [w271 w273] -> w225
      frame No Error {
      }
      frame Error {
        n114 = call "QMH_UI_Control_EnQueue.vi"("Last ?"=FALSE, "Command"=QMH_UI_Command."UI Exit", "UI Queue"=w276) -> ("error out"=w273:errorcluster)  [unwired: 7 in, 1 out]
      }
    }
  }
  n115 = Unregister For Events(event registration refnum=w14, error in=w15) -> (error out=w11:errorcluster)
  n116 = Destroy User Event(user event=w12, error in=w11) -> (error out=w10:errorcluster)
  n117 = Merge Errors(w10, w13, w3) -> (w6:errorcluster)
  n118 = property on="Property Node" class="App"(error in=w6) -> (error out=w9:errorcluster, "App.Kind"=w8:T28)  [unwired: 1 in, 1 out]
  n119 = call <vilib>:"Simple Error Handler.vi"("error in (no error)"=w9) -> ("error out"=w7:errorcluster)  [unwired: 4 in, 4 out]
  n120 = case shown="Par défaut" w8 {
    tunnel: w7 -> [_ _]
    frame Default {
    }
    frame "Run Time System" {
      n121 = Quit LabVIEW() -> ()  [unwired: 1 in]
    }
  }
